vi "SngJntArmSim_Pack_Simulation_Params.vi"(8 "SimulateGravity":bool=TRUE, 9 "Pos Sim StdDev Rad":dbl=0.09, 10 "MaxAngle_Rad":dbl, 11 "MinAngle_Rad":dbl) -> (3 "SngJntArmSim_Simulation _Params":T1 {"Measurment StdDev" format="%#_13g"})   [LabVIEW 2019, in "Trajectory_Library.lvlib"]
doc: "Pack simulation parameters used by the Single Jointed Arm Simulation Execute routine.\n\nInputs:\n - Min Angle -- double -- Minimum physical arm angle (radians)\n - Max Angle -- double -- Maximum physical arm angle (radians)\n - Pos Sim Std Dev -- double -- Standard deviation for the arm position (radians Default: 0.09)\n - SimulateGravity -- boolean -- Simulate gravity (Default: True)\n\nOutputs:\n - SngJntArm Sim Simulation -- cluster -- Packed data for Execute function"
uses:
  Trajectory_Library.lvlib
  TypeDef/SINGLE_JOINT_ARM_SIM_SIMULATION_PARAMS.ctl
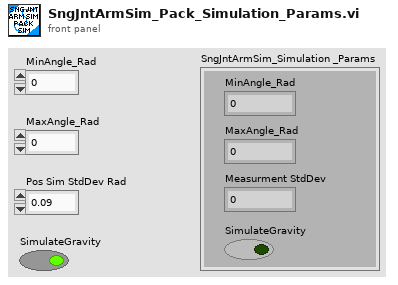
[diagram p1: front panel]
types:
  T1 = typedef "Trajectory_Library.lvlib/SINGLE_JOINT_ARM_SIM_SIMULATION_PARAMS.ctl" = cluster{"MinAngle_Rad":dbl, "MaxAngle_Rad":dbl, "Measurment StdDev":dbl, "SimulateGravity":bool}
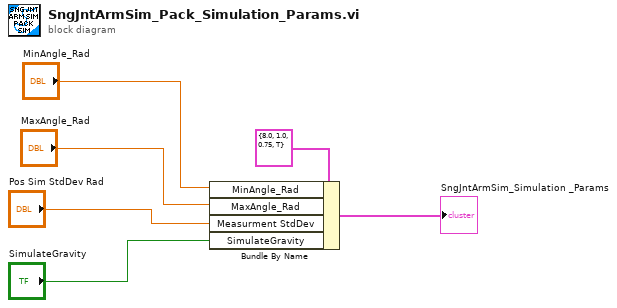
[diagram p0: block diagram]
diagram:
  n1 = Bundle By Name(cluster=T1 {"MinAngle_Rad"=8.0, "MaxAngle_Rad"=1.0, "Measurment StdDev"=0.75, "SimulateGravity"=TRUE} ("SngJntArmSim_Simulation _Params"), "MinAngle_Rad"="MinAngle_Rad", "MaxAngle_Rad"="MaxAngle_Rad", "Measurment StdDev"="Pos Sim StdDev Rad", "SimulateGravity"="SimulateGravity") -> (→"SngJntArmSim_Simulation _Params":T1)
